vi "PLC Status.vi"(8 "error in (no error)":errorcluster, 10 "PLC Status":bool, 11 "UserInterface in":refnum<class "UserInterface.lvclass">) -> (0 "error out":errorcluster, 3 "UserInterface out":refnum<class "UserInterface.lvclass">)   [LabVIEW 2022 SP3, in "UserInterface.lvlib" / "UserInterface.lvclass"]
uses:
  UserInterface.lvclass
  UserInterface.lvclass/UserInterface.ctl
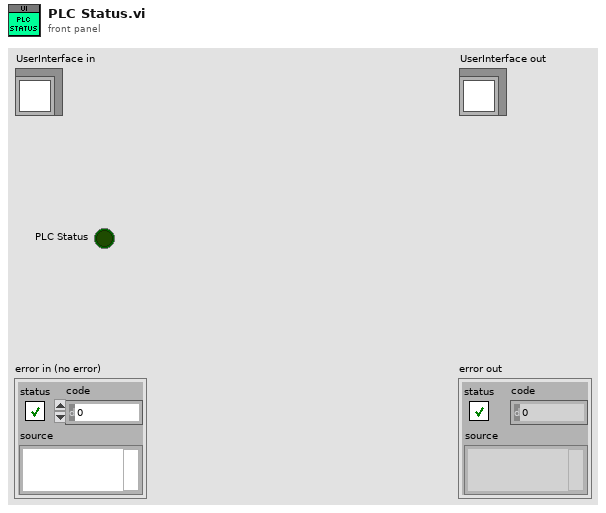
[diagram p1: front panel]
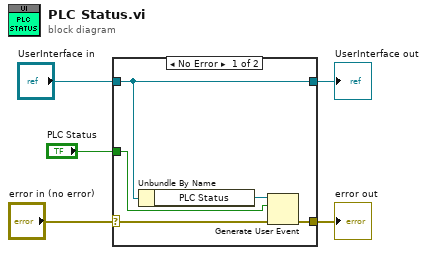
[diagram p0: block diagram]
diagram:
  n1 = case shown="No Error" "error in (no error)" {
    selector: "error in (no error)" -> [w7 w12]
    tunnel: [w6 w12] -> w4
    tunnel: [w9 w11] -> w2
    tunnel: "UserInterface in" -> [w9 w11]
    tunnel: "PLC Status" -> [w8 _]
    frame No Error {
      n2 = Unbundle By Name(w9) -> ("PLC Status"=w10:refnum<user-event>)
      n3 = Generate User Event(user event=w10, event data cluster=w8, error in=w7) -> (error out=w6:errorcluster)  [unwired: 1 in, 1 out]
    }
    frame Error {
    }
  }
  "error out" <- w4
  "UserInterface out" <- w2
